vi "Lighting Test Software Lightshow.vi"() -> ()   [LabVIEW 2020]
panel:
  in  "Tab Control":enum32{"Map", "Settings", "LightShow"}(tab)=enum."LightShow"
  in  "Slide":dbl(slide)=0.7342857142857143 scale=0.0..1.0
  in  "Array 3":cluster{"Color Box":u32, "Slide":dbl}[][](array[cluster])=[[{"Color Box"=12303291, "Slide"=10.0}, {"Color Box"=12303291, "Slide"=10.0}, {"Color Box"=12303291, "Slide"=10.0}, {"Color Box"=12303291, "Slide"=10.0}, {"Color Box"=12303291, "Slide"=10.0}, {"Color Box"=12303291, "Slide"=10.0}], [{"Color Box"=12303291, "Slide"=10.0}, {"Color Box"=12303291, "Slide"=10.0}, {"Color Box"=12303291, "Slide"=10.0}, {"Color Box"=12303291, "Slide"=10.0}, {"Color Box"=12303291, "Slide"=10.0}, {"Color Box"=12303291, "Slide"=10.0}], [{"Color Box"=12303291, "Slide"=10.0}, {"Color Box"=12303291, "Slide"=10.0}, {"Color Box"=12303291, "Slide"=10.0}, {"Color Box"=12303291, "Slide"=10.0}, {"Color Box"=12303291, "Slide"=10.0}, {"Color Box"=12303291, "Slide"=10.0}], [{"Color Box"=12303291, "Slide"=10.0}, {"Color Box"=12303291, "Slide"=10.0}, {"Color Box"=12303291, "Slide"=10.0}, {"Color Box"=12303291, "Slide"=10.0}, {"Color Box"=0, "Slide"=0.0}, {"Color Box"=0, "Slide"=0.0}], [{"Color Box"=12303291, "Slide"=10.0}, {"Color Box"=12303291, "Slide"=10.0}, {"Color Box"=0, "Slide"=0.0}, {"Color Box"=12303291, "Slide"=10.0}, {"Color Box"=0, "Slide"=0.0}, {"Color Box"=0, "Slide"=0.0}], [{"Color Box"=0, "Slide"=0.0}, {"Color Box"=0, "Slide"=0.0}, {"Color Box"=12303291, "Slide"=10.0}, {"Color Box"=0, "Slide"=0.0}, {"Color Box"=0, "Slide"=0.0}, {"Color Box"=0, "Slide"=0.0}]] {"Slide" min=0.0 max=10.0 scale=-1.0..11.0 scale format="%_1g"}
  in  "Save Config":bool
  in  "Load Config":bool
  in  "Index":cluster{"Numeric":i32}[][](array[cluster])=[[{"Numeric"=3}, {"Numeric"=9}, {"Numeric"=2}, {"Numeric"=8}, {"Numeric"=19}, {"Numeric"=23}], [{"Numeric"=1}, {"Numeric"=11}, {"Numeric"=0}, {"Numeric"=10}, {"Numeric"=17}, {"Numeric"=21}], [{"Numeric"=5}, {"Numeric"=13}, {"Numeric"=4}, {"Numeric"=14}, {"Numeric"=27}, {"Numeric"=25}], [{"Numeric"=7}, {"Numeric"=15}, {"Numeric"=6}, {"Numeric"=12}, {"Numeric"=26}, {"Numeric"=24}], [{"Numeric"=29}, {"Numeric"=31}, {"Numeric"=-1}, {"Numeric"=18}, {"Numeric"=-1}, {"Numeric"=22}], [{"Numeric"=30}, {"Numeric"=-1}, {"Numeric"=16}, {"Numeric"=-1}, {"Numeric"=-1}, {"Numeric"=-1}]]
  in  "physical channels":refnum<k21>="Dev0/Ao0:15"
  in  "physical channels 2":refnum<k21>="Dev1/Ao0:15"
  out "error out":errorcluster
  out "specific error cleared?":bool
  in  "Choose Test":string(combo)="Test 1"
  out "Waveform Chart":dbl(graph)
  in  "LightShow":bool
  in  "OK":bool
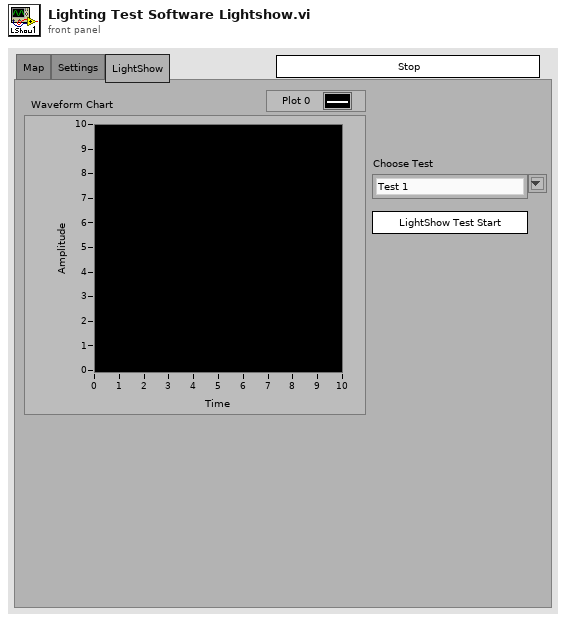
[diagram p1: front panel]
types:
  T1 = enum32{"invalid app kind", "Development System", "Run Time System", "Student Edition", "Embedded LabVIEW", "Evaluation", "Custom"}
  T2 = enum32{"Invalid", "Standard", "Closed", "Hidden", "Minimized", "Maximized"}
  T3 = cluster{"Slide Value Low":dbl, "Slide Value High":dbl}
  T4 = cluster{"Core":cluster{"Current VI Reference":refnum<vi>, "Close Panel on Exit?":bool}, "Your Boolean data":bool, "Slide Value":dbl, "Current Test":string, "Test Info":cluster{"Slide Value Low":dbl, "Slide Value High":dbl}}
  T5 = cluster{"Current VI Reference":refnum<vi>, "Close Panel on Exit?":bool}
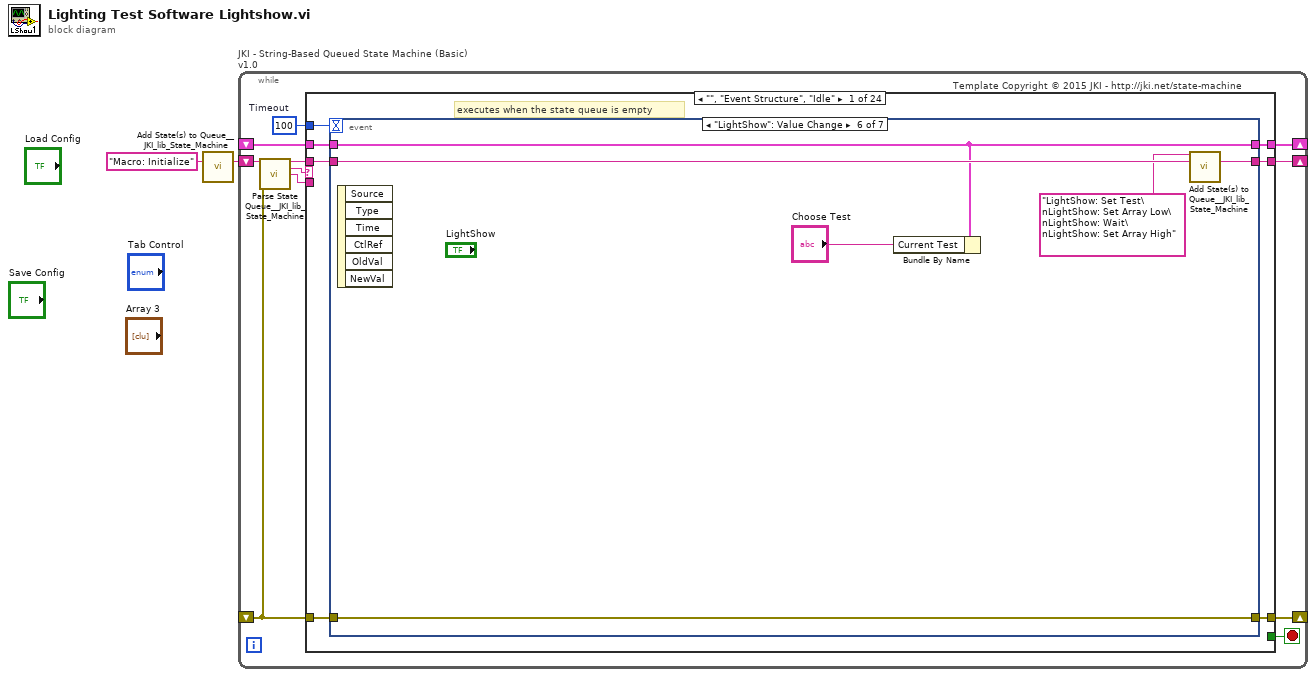
[diagram p0: block diagram]
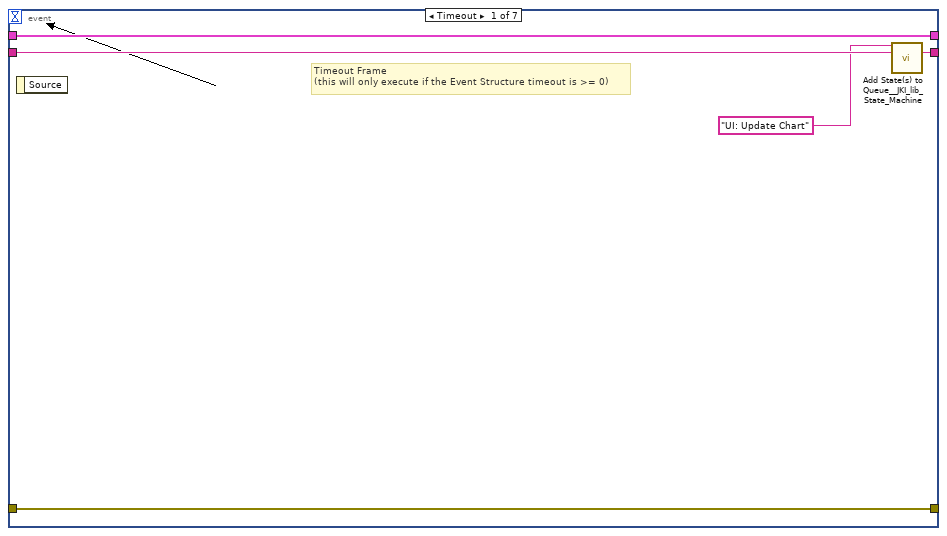
[diagram p2: hidden frame]
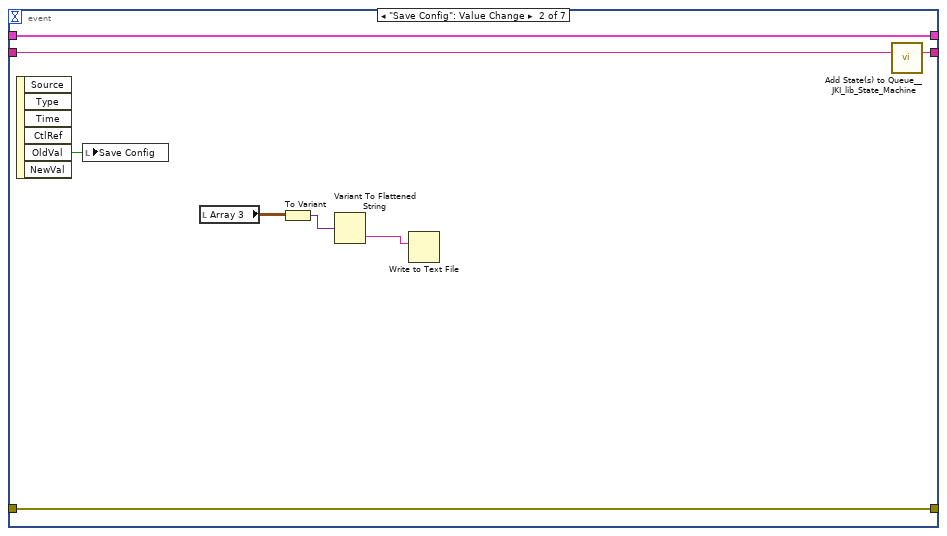
[diagram p3: hidden frame]
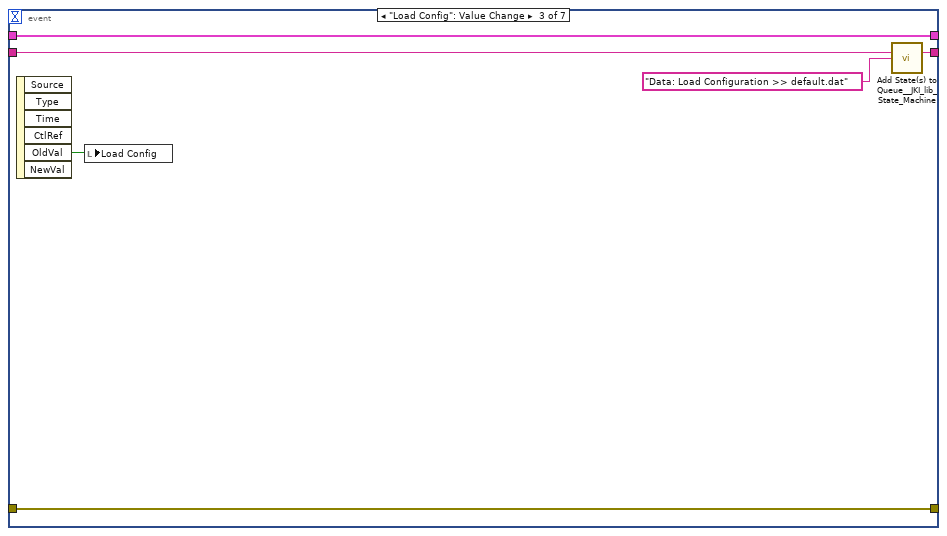
[diagram p4: hidden frame]
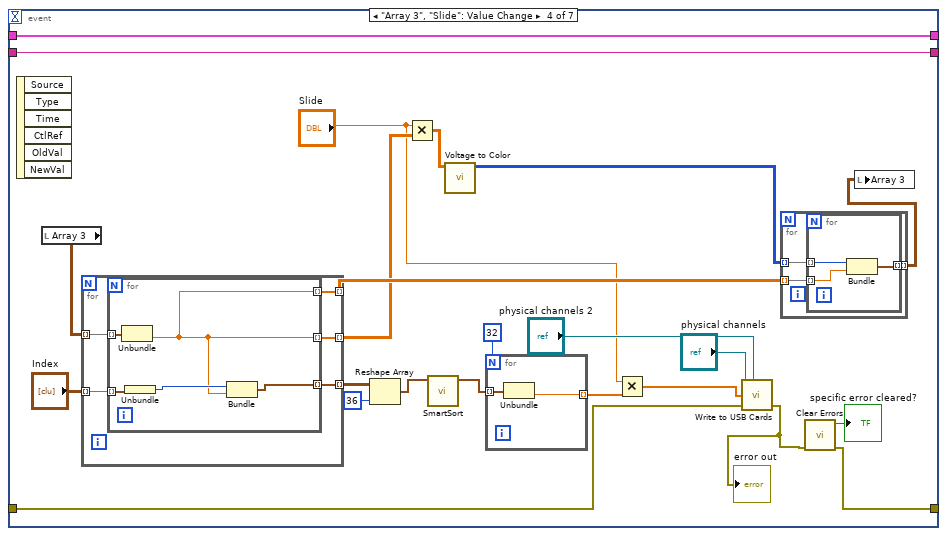
[diagram p5: hidden frame]
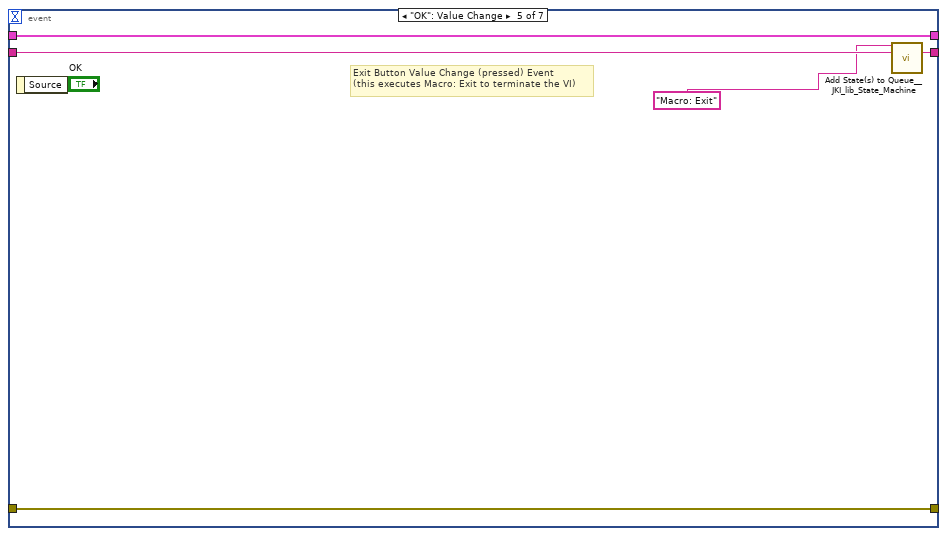
[diagram p6: hidden frame]
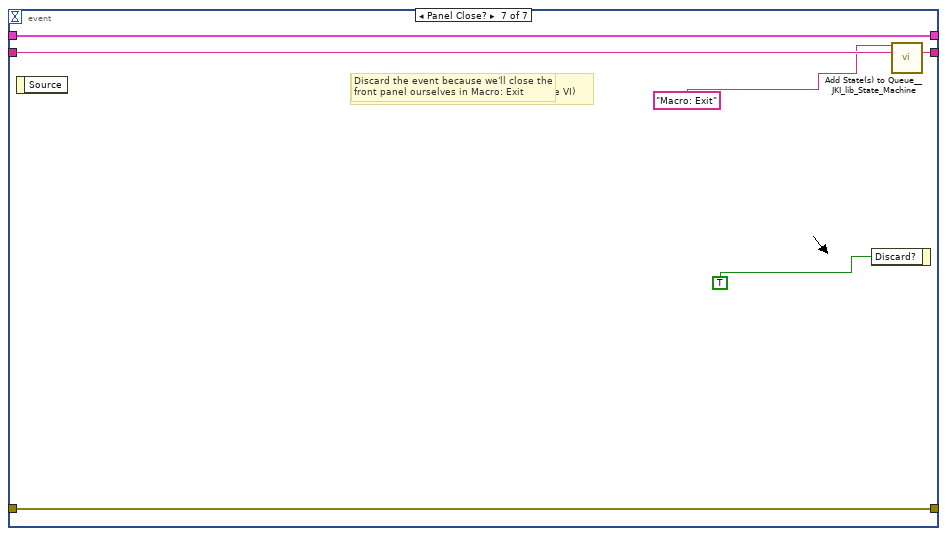
[diagram p7: hidden frame]
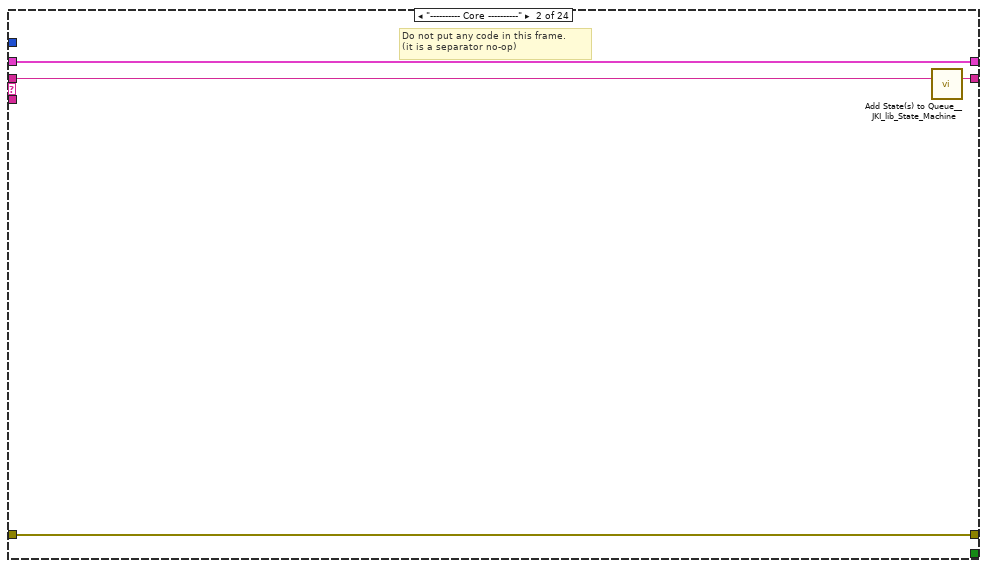
[diagram p8: hidden frame]
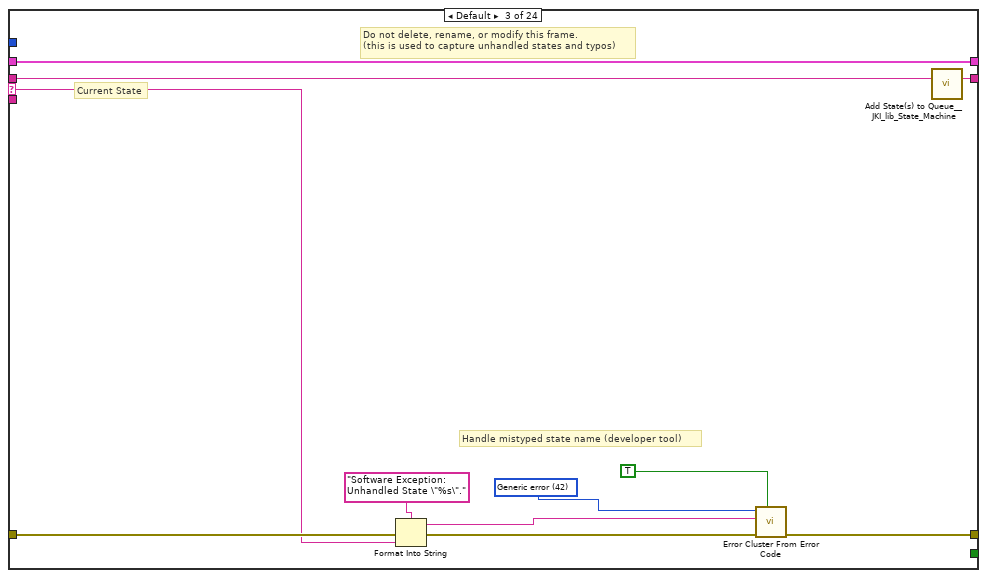
[diagram p9: hidden frame]
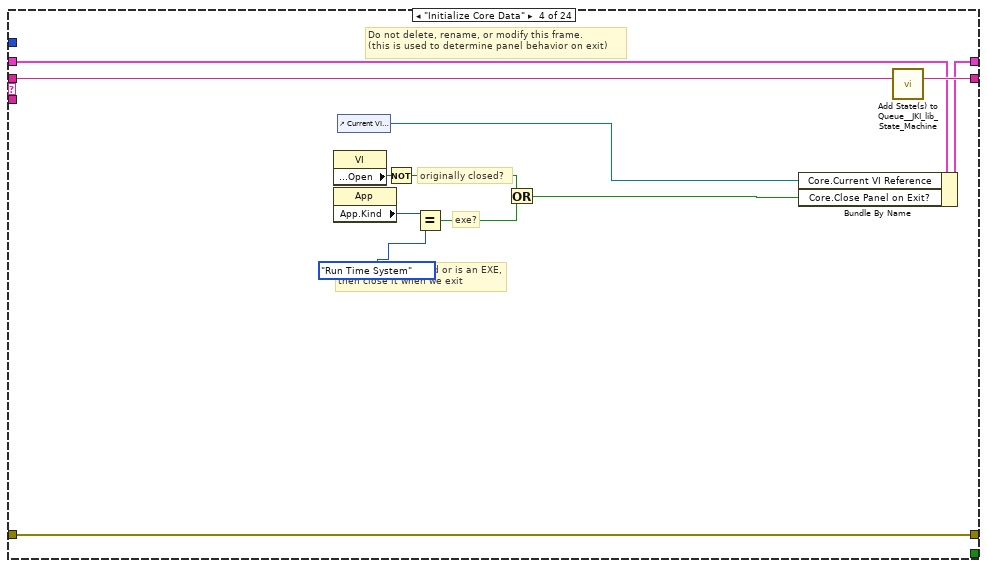
[diagram p10: hidden frame]
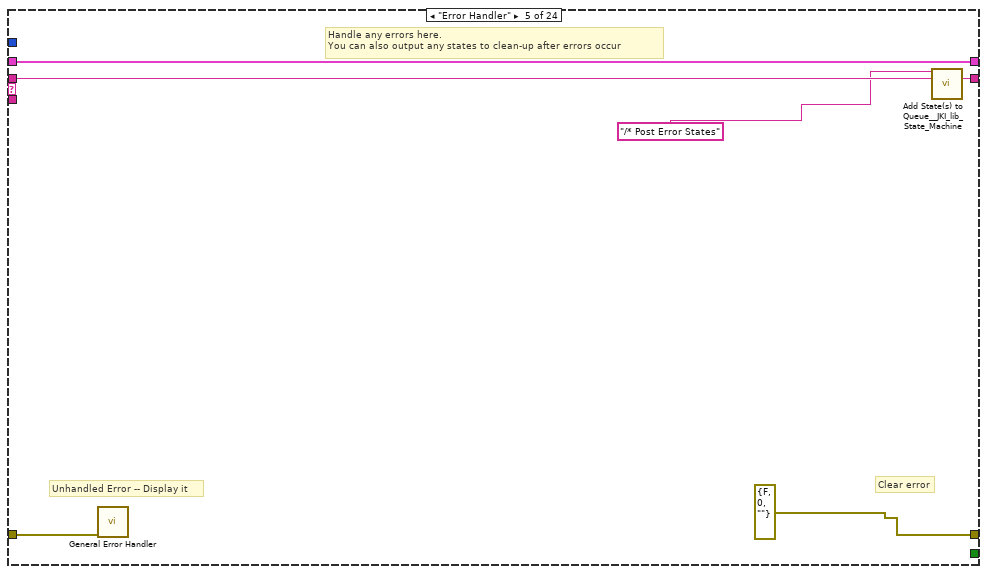
[diagram p11: hidden frame]
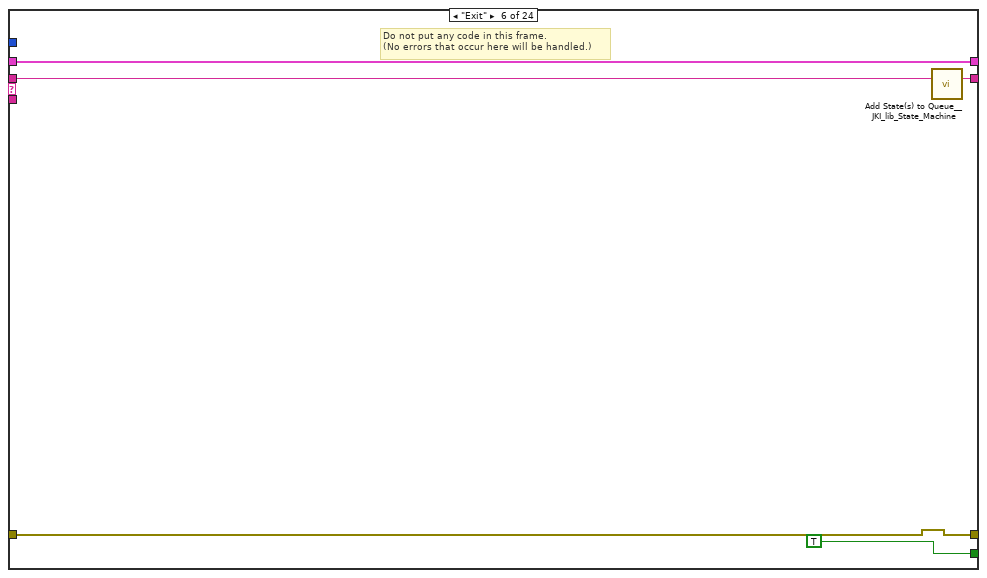
[diagram p12: hidden frame]
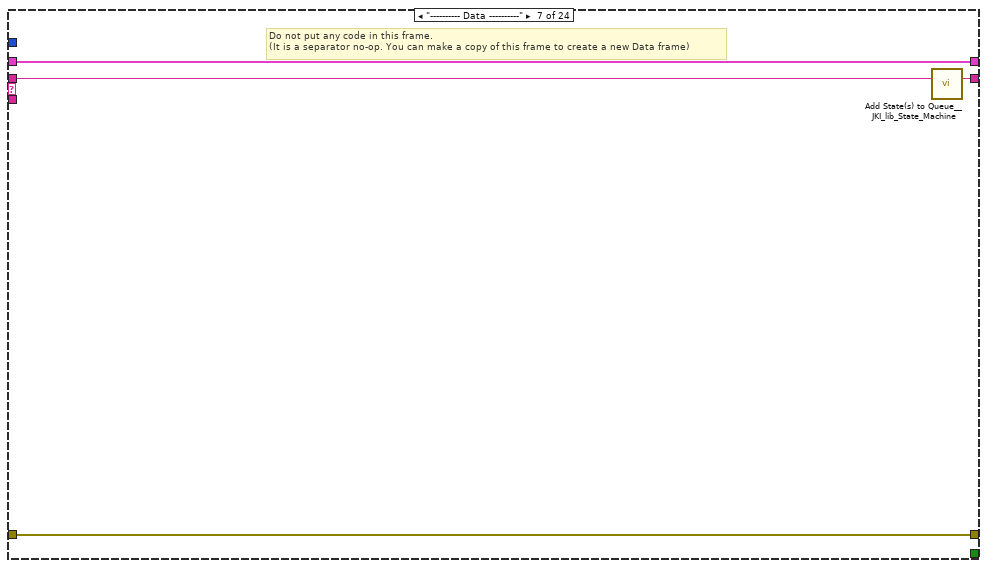
[diagram p13: hidden frame]
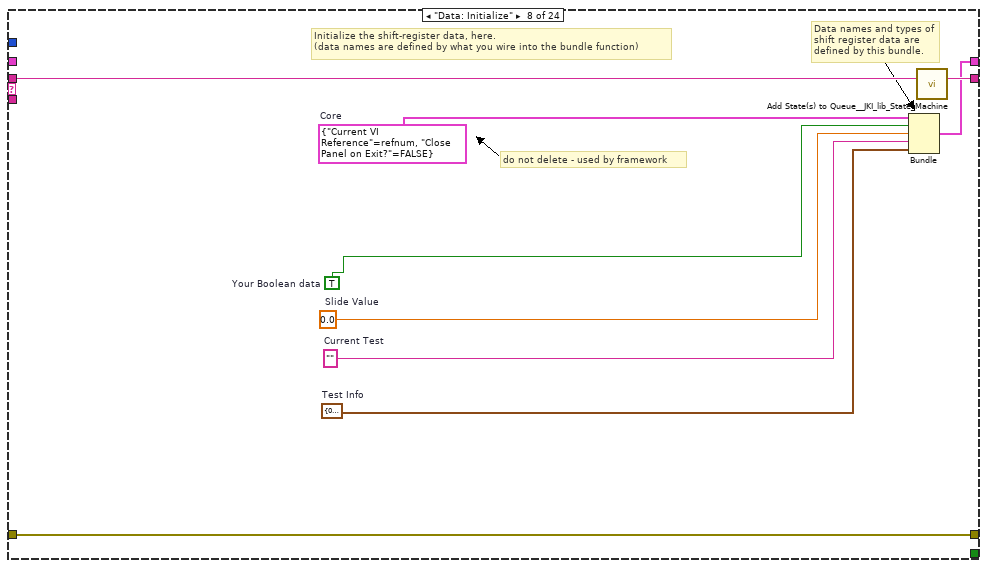
[diagram p14: hidden frame]
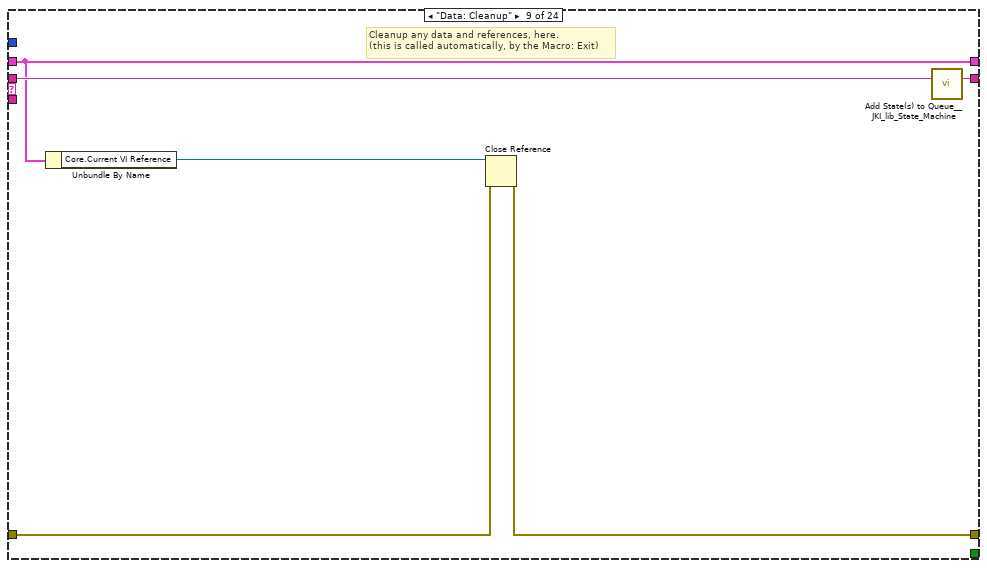
[diagram p15: hidden frame]
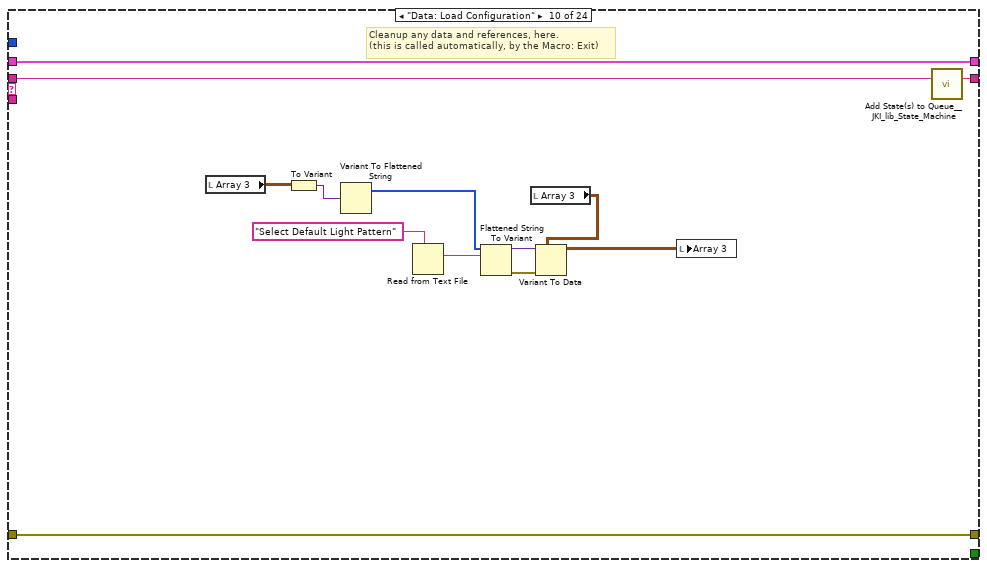
[diagram p16: hidden frame]
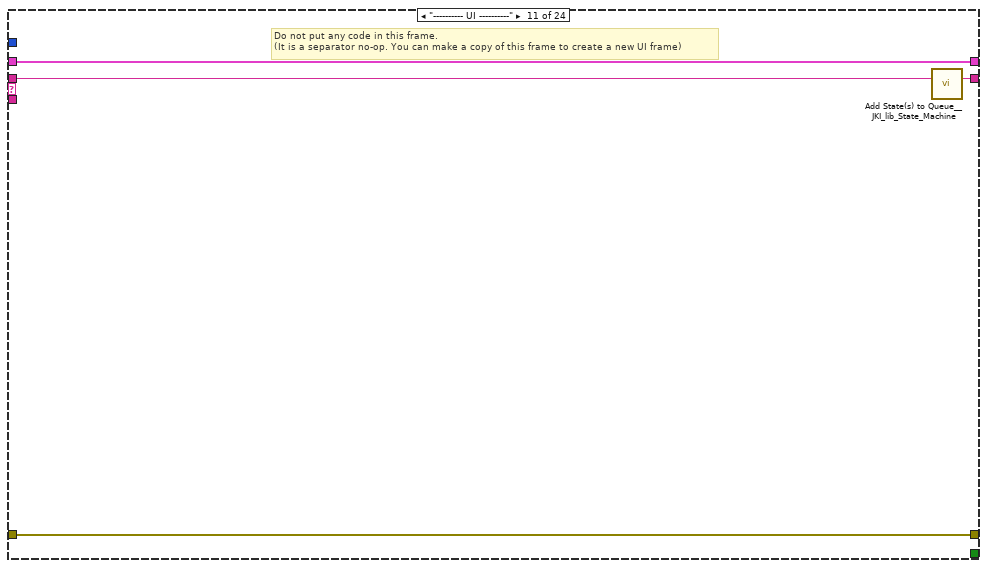
[diagram p17: hidden frame]
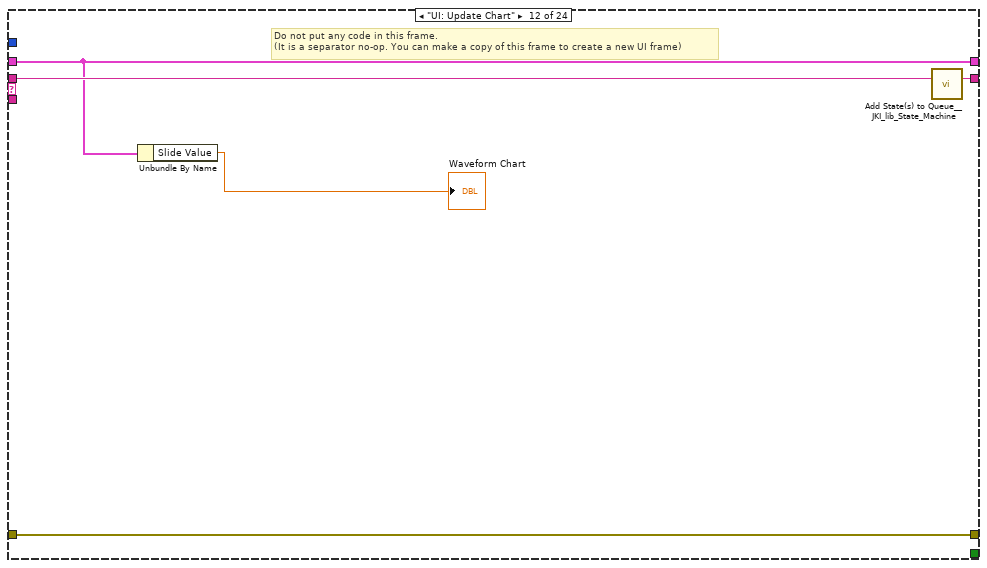
[diagram p18: hidden frame]
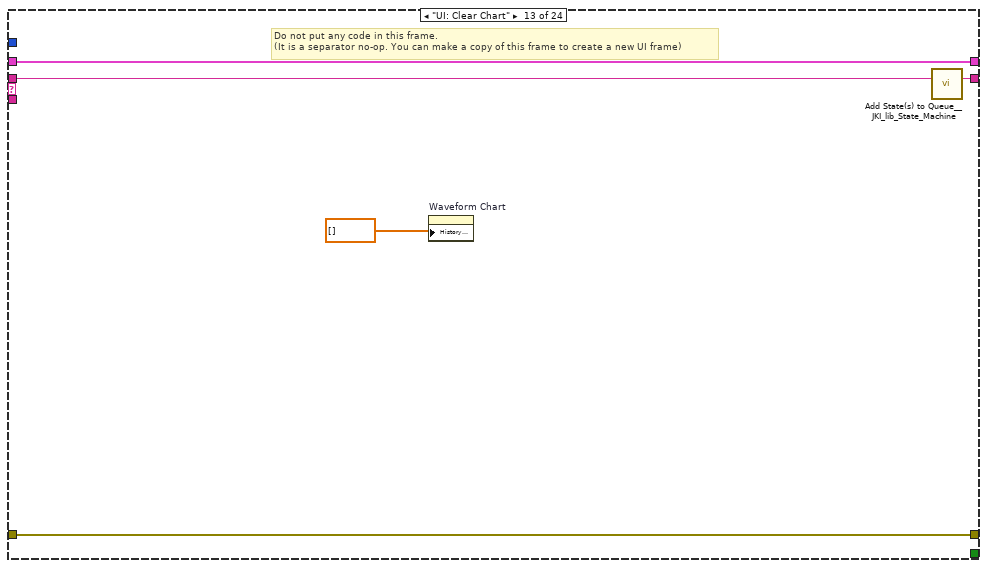
[diagram p19: hidden frame]
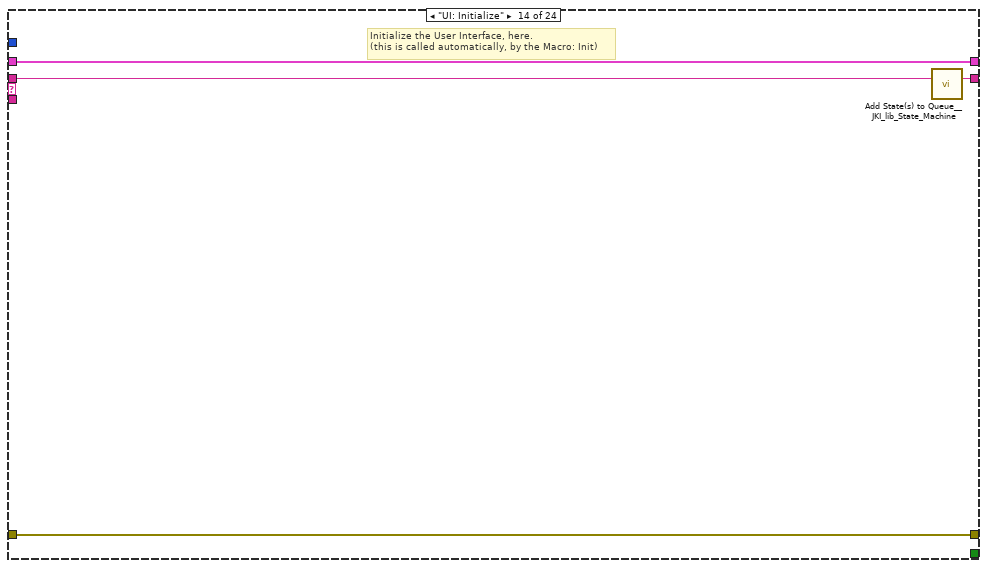
[diagram p20: hidden frame]
diagram:
  n1 = call <vilib>:"Add State(s) to Queue__JKI_lib_State_Machine.vi"("State(s) in (\"\")"="Macro: Initialize") -> ("States Out"=w2:string)  [unwired: 14 in]
  n2 = while "JKI - String-Based Queued State Machine (Basic) v1.0" {
    shift-right: [w6] -> _
    shift-left: _ -> [w5]
    shift-right: [w9] -> _
    shift-left: _ -> [w3]
    shift-right: [w8] -> _
    shift-left: w2 -> [w10]
    stop <- w7 stop-if-true
    w4 = 100  # Timeout
    # "Template Copyright © 2015 JKI - http://jki.net/state-machine"
    n3 = call <vilib>:"Parse State Queue__JKI_lib_State_Machine.vi"("State Queue"=w10, "Error In (no error)"=w3) -> ("Remaining States"=w12:string, "Current State"=w13:string, "Arguments"=w11:string)  [unwired: 11 in]
    n4 = case shown="\"\", \"Event Structure\", \"Idle\"" w13 {
      selector: w13 -> [_ _ w102 _ _ _ _ _ _ _ _ _ _ _ _ _ _ _ _ _ _ _ _ _]
      tunnel: w12 -> [w20 w101 w106 w124 w130 w135 w139 w148 w154 w167 w171 w176 w181 w185 w191 w202 w228 w233 w243 w247 w255 w262 w290 w333]
      tunnel: w11 -> [_ _ _ _ _ _ _ _ _ _ _ _ _ _ w186 w196 _ _ _ _ _ _ _ _]
      tunnel: w5 -> [w18 w98 w104 w115 w127 w132 w136 _ w149 w165 w168 w173 w178 w183 w189 w198 w225 w230 w240 w244 w253 w257 w268 w311]
      tunnel: [w17 w99 w108 w121 errorcluster {"status"=FALSE, "code"=0, "source"=""} ("error out") w131 w137 w143 w150 w164 w169 w174 w179 w182 w187 w199 w226 w231 w241 w245 w251 w260 w269 w312] -> w9
      tunnel: w3 -> [w16 w99 w107 w121 w126 w131 w137 w143 w151 w164 w169 w174 w179 w182 w188 w200 w226 w231 w241 w245 w252 w260 w270 w313]
      tunnel: [w19 w100 w105 w123 w129 w134 w138 w147 w153 w166 w170 w175 w180 w184 w190 w201 w227 w232 w242 w246 w254 w261 w289 w332] -> w8
      tunnel: [_ _ _ _ _ TRUE _ _ _ _ _ _ _ _ _ _ _ _ _ _ _ _ _ _] -> w7
      tunnel: [w15 w98 w104 w122 w127 w132 w136 w146 w149 w165 w168 w173 w178 w183 w189 w198 w225 w230 w240 w244 w253 w257 w267 w310] -> w6
      tunnel: w4 -> [w14 _ _ _ _ _ _ _ _ _ _ _ _ _ _ _ _ _ _ _ _ _ _ _]
      frame "", "Event Structure", "Idle" {
        # "executes when the state queue is empty"
        n5 = event shown="[5] \"LightShow\": Value Change" {
          selector: _ -> [_ _ _ _ _ _ _]
          dyn-events: _ -> [_ _ _ _ _ _ _]
          timeout: w14 -> [_ _ _ _ _ _ _]
          tunnel: w20 -> [w25 w33 w39 w61 w85 w90 w97]
          tunnel: [w24 w32 w38 w61 w84 w91 w96] -> w19
          tunnel: w18 -> [w22 w30 w36 w62 w82 w88 w94]
          tunnel: [w23 w31 w37 w47 w83 w86 w95] -> w17
          tunnel: w16 -> [w23 w31 w37 w48 w83 w86 w95]
          tunnel: [w22 w30 w36 w62 w82 w88 w94] -> w15
          event Timeout {
            # "Timeout Frame\n(this will only execute if the Event Structure timeout is >= 0)"
            n6 = event-data() -> ()  [unwired: 1 in, 1 out]
            n7 = call <vilib>:"Add State(s) to Queue__JKI_lib_State_Machine.vi"("State(s) in Front (\"\")"="UI: Update Chart" ("State(s) in Front (\"\")"), "State(s) in (\"\")"=w25) -> ("States Out"=w24:string)  [unwired: 13 in]
          }
          event "Save Config": Value Change {
            n8 = event-data() -> ("OldVal"=w26:bool)  [unwired: 1 in, 5 out]
            n9 = local write "Save Config"(w26) -> ()
            n10 = local read "Array 3"() -> (w29:cluster{"Color Box":u32, "Slide":dbl}[][])
            n11 = To Variant(anything=w29) -> (Variant=w28:variant)
            n12 = Variant To Flattened String(Variant=w28) -> (data string=w27:string)  [unwired: 1 out]
            n13 = Write to Text File(text=w27) -> ()  [unwired: 3 in, 3 out]
            n14 = call <vilib>:"Add State(s) to Queue__JKI_lib_State_Machine.vi"("State(s) in (\"\")"=w33) -> ("States Out"=w32:string)  [unwired: 14 in]
          }
          event "Load Config": Value Change {
            n15 = event-data() -> ("OldVal"=w35:bool)  [unwired: 1 in, 5 out]
            n16 = local write "Load Config"(w35) -> ()
            n17 = call <vilib>:"Add State(s) to Queue__JKI_lib_State_Machine.vi"("State(s) in (\"\")"=w39, "State(s) at Back (\"\")"="Data: Load Configuration >> default.dat") -> ("States Out"=w38:string)  [unwired: 13 in]
          }
          event "Array 3", "Slide": Value Change {
            n18 = event-data() -> ()  [unwired: 1 in, 6 out]
            n19 = local read "Array 3"() -> (w60:cluster{"Color Box":u32, "Slide":dbl}[][])
            n20 = for {
              tunnel: w60 -> [w75] mode=indexing
              tunnel: [w74] -> w44 mode=indexing
              tunnel: [w73] -> w57 mode=indexing
              tunnel: "Index" -> [w72] mode=indexing
              tunnel: [w71] -> w55 mode=indexing
              n21 = for {
                tunnel: w75 -> [w80] mode=indexing
                tunnel: [w77] -> w74 mode=indexing
                tunnel: [w77] -> w73 mode=indexing
                tunnel: w72 -> [w79] mode=indexing
                tunnel: [w76] -> w71 mode=indexing
                n22 = Unbundle(w80) -> ("Slide"=w77:dbl)  [unwired: 1 out]
                n23 = Unbundle(w79) -> ("Numeric"=w78:i32)
                n24 = Bundle("Numeric"=w78, "Slide"=w77) -> (w76:cluster{"Numeric":i32, "Slide":dbl})  [unwired: 1 in]
              }
            }
            n25 = Reshape Array(w55, 36 ("dimension size")) -> (w53:cluster{"Numeric":i32, "Slide":dbl}[])
            n26 = Multiply(x="Slide", y=w44) -> (x*y=w43:dbl[][])
            n27 = call "SmartSort.vi"("Array in"=w53) -> ("Array out"=w52:cluster{"Numeric":i32, "Slide":dbl}[])  [unwired: 10 in]
            n28 = call "Voltage to Color.vi"("Array in"=w43) -> ("Array out"=w58:u32[][])  [unwired: 10 in]
            n29 = for {
              N: 32 -> [_]
              tunnel: w52 -> [w64] mode=indexing
              tunnel: [w63] -> w42 mode=indexing
              n30 = Unbundle(w64) -> ("Slide"=w63:dbl)  [unwired: 1 out]
            }
            n31 = Multiply(x="Slide", y=w42) -> (x*y=w40:dbl[])
            n32 = call "Write to USB Cards.vi"("physical channels"="physical channels", "physical channels 2"="physical channels 2", "Array"=w40, "error in"=w48) -> ("error out"=w45:errorcluster)  [unwired: 5 in]
            "error out" <- w45
            n33 = for {
              tunnel: [w67] -> w59 mode=indexing
              tunnel: w58 -> [w66] mode=indexing
              tunnel: w57 -> [w65] mode=indexing
              n34 = for {
                tunnel: [w70] -> w67 mode=indexing
                tunnel: w66 -> [w69] mode=indexing
                tunnel: w65 -> [w68] mode=indexing
                n35 = Bundle(w69, "Slide"=w68) -> (w70:cluster{u32, "Slide":dbl})  [unwired: 1 in]
              }
            }
            n36 = call <vilib>:"Clear Errors.vi"("error in (no error)"=w45) -> ("error out"=w47:errorcluster, "specific error cleared?"=→"specific error cleared?":bool)  [unwired: 5 in]
            n37 = local write "Array 3"(w59) -> ()
          }
          event "OK": Value Change {
            # "Exit Button Value Change (pressed) Event\n(this executes Macro: Exit to terminate the VI)"
            n38 = event-data() -> ()  [unwired: 1 in, 1 out]
            n39 = call <vilib>:"Add State(s) to Queue__JKI_lib_State_Machine.vi"("State(s) in Front (\"\")"="Macro: Exit", "State(s) in (\"\")"=w85) -> ("States Out"=w84:string)  [unwired: 13 in]
          }
          event "LightShow": Value Change {
            n40 = event-data() -> ()  [unwired: 1 in, 6 out]
            n41 = Bundle By Name(cluster=w88, "Current Test"="Choose Test") -> ()  [unwired: 1 out]
            n42 = call <vilib>:"Add State(s) to Queue__JKI_lib_State_Machine.vi"("State(s) in Front (\"\")"="LightShow: Set Test\nLightShow: Set Array Low\nLightShow: Wait\nLightShow: Set Array High" ("State(s) in Front (\"\")"), "State(s) in (\"\")"=w90) -> ("States Out"=w91:string)  [unwired: 13 in]
          }
          event Panel Close? {
            # "Discard the event because we'll close the front panel ourselves in Macro: Exit"
            # "Close Panel button (pressed) Event\n(this executes Macro: Exit to terminate the VI)"
            n43 = event-data() -> ()  [unwired: 1 in, 1 out]
            n44 = event-data("Discard?"=TRUE) -> ()  [unwired: 1 in, 1 out]
            n45 = call <vilib>:"Add State(s) to Queue__JKI_lib_State_Machine.vi"("State(s) in Front (\"\")"="Macro: Exit", "State(s) in (\"\")"=w97) -> ("States Out"=w96:string)  [unwired: 13 in]
          }
        }
      }
      frame "---------- Core ----------" {
        # "Do not put any code in this frame.\n(it is a separator no-op)"
        n46 = call <vilib>:"Add State(s) to Queue__JKI_lib_State_Machine.vi"("State(s) in (\"\")"=w101) -> ("States Out"=w100:string)  [unwired: 14 in]
      }
      frame Default {
        w111 = 42 items=["No error", "Argument error", "Memory is full", "Out of zone", "End of file", "File already open", "Generic file I/O error", "File not found", "File permission error", "Disk is full", "Duplicate path", "Too many files open", "System feature not enabled", "Resource file not found", "Cannot add resource", "Resource not found", "Image not found", "Image memory error", "Pen does not exist", "Config type invalid", "Config token not found", "Config parse error", "Config memory error", "Bad external code format", "Bad external code offset", "External code not present", "Null window", "Destroy window error", "Null menu", "Print aborted", "Bad print record", "Print driver error", "Windows error during printing", "Memory error during printing", "Print dialog error", "Generic print error", "Invalid device refnum", "Device not found", "Device parameter error", "Device unit error", "Cannot open device", "Device call aborted", "Generic error", "Cancelled by user", "Object ID too low", "Object ID too high", "Object not in heap", "Unknown heap", "Unknown object (invalid DefProc)", "Unknown object (DefProc not in table)", "Message out of range", "Invalid (null) method", "Unknown message", "Manager call not supported", "Bad address", "Network operation in progress", "Network operation timed out", "Connection is busy", "Network attribute not supported", "Network error", "Address in use", "System out of memory", "Connection aborted", "Connection refused", "Not connected", "Already connected", "Connection closed", "Initialization error (interapplication manager)", "Bad occurrence", "Wait on unbound occurrence handler", "Occurrence queue overflow", "Datalog type conflict", "Unused", "Unrecognized type (interapplication manager)", "Memory corrupt", "Failed to make temporary DLL", "Old CIN version", "Drag socket not found", "Failed to load drop-object", "Failed to register OLE object", "Failed to release OLE object", "Format specifier type mismatch", "Unknown format specifier", "Too few format specifiers", "Too many format specifiers", "Scan failed", "Newer CIN version", "Error converting to variant", "Runtime menu error", "Password tampered", "Variant attribute not found", "Incompatible variant data type", "Event data is not available", "Event Store is not present", "Occurrence is not found", "Event Queue is not created", "Event info is not available", "Refnum passed is NULL", "Error retrieving Class GUID", "Error retrieving CoClass GUID", "Error retrieving TypeLib GUID.", "Bad built application magic bytes.", "Specific driver is different from the specific driver associated with the Logical Name.", "There is no session opened to the class driver.", "Max Error", "MAX - Error with config objects", "MAX - Error loading configuration", "MAX - Group not supported"]
        # "Current State"
        # "Do not delete, rename, or modify this frame.\n(this is used to capture unhandled states and typos)"
        # "Handle mistyped state name (developer tool)"
        n47 = Format Into String(format string="Software Exception: Unhandled State \"%s\"." ("message"), error in=w107, w102) -> (resulting string=w110:string, error out=w109:errorcluster)  [unwired: 1 in]
        n48 = call <vilib>:"Error Cluster From Error Code.vi"("show call chain? (False)"=TRUE, "error in (no error)"=w109, "error message (\"\")"=w110, "error code (0)"=w111) -> ("error out"=w108:errorcluster)  [unwired: 5 in]
        n49 = call <vilib>:"Add State(s) to Queue__JKI_lib_State_Machine.vi"("State(s) in (\"\")"=w106) -> ("States Out"=w105:string)  [unwired: 14 in]
      }
      frame "Initialize Core Data" {
        # "Do not delete, rename, or modify this frame.\n(this is used to determine panel behavior on exit)"
        # "originally closed?"
        # "exe?"
        # "If panel starts closed or is an EXE, then close it when we exit"
        n50 = property class="VI"() -> ("Front Panel.Open"=w120:bool)  [unwired: 2 in, 2 out]
        n51 = property class="App"() -> ("App.Kind"=w119:T1)  [unwired: 2 in, 2 out]
        n52 = control-ref of="Current VI Reference"() -> (w113:refnum<vi>)
        n53 = Not(x=w120) -> (.not. x?=w117:bool)
        n54 = Equal?(x=w119, y=T1."Run Time System" ("Application:Kind")) -> (x = y?=w116:bool)
        n55 = Or(x=w117, y=w116) -> (x .or. y?=w114:bool)
        n56 = Bundle By Name(cluster=w115, "Core.Current VI Reference"=w113, "Core.Close Panel on Exit?"=w114) -> (w122:T4)
        n57 = call <vilib>:"Add State(s) to Queue__JKI_lib_State_Machine.vi"("State(s) in (\"\")"=w124) -> ("States Out"=w123:string)  [unwired: 14 in]
      }
      frame "Error Handler" {
        # "Unhandled Error -- Display it"
        # "Handle any errors here.\nYou can also output any states to clean-up after errors occur"
        # "Clear error"
        n58 = call <vilib>:"General Error Handler.vi"("error in (no error)"=w126) -> ()  [unwired: 10 in, 5 out]
        n59 = call <vilib>:"Add State(s) to Queue__JKI_lib_State_Machine.vi"("State(s) in Front (\"\")"="/* Post Error States", "State(s) in (\"\")"=w130) -> ("States Out"=w129:string)  [unwired: 13 in]
      }
      frame "Exit" {
        # "Do not put any code in this frame.\n(No errors that occur here will be handled.)"
        n60 = call <vilib>:"Add State(s) to Queue__JKI_lib_State_Machine.vi"("State(s) in (\"\")"=w135) -> ("States Out"=w134:string)  [unwired: 14 in]
      }
      frame "---------- Data ----------" {
        # "Do not put any code in this frame.\n(It is a separator no-op. You can make a copy of this frame to create a new Data frame)"
        n61 = call <vilib>:"Add State(s) to Queue__JKI_lib_State_Machine.vi"("State(s) in (\"\")"=w139) -> ("States Out"=w138:string)  [unwired: 14 in]
      }
      frame "Data: Initialize" {
        w140 = T3 {"Slide Value Low"=0.0, "Slide Value High"=0.0}  # Test Info
        w141 = ""  # Current Test
        w142 = 0.0  # Slide Value
        w144 = T5 {"Current VI Reference"=refnum, "Close Panel on Exit?"=FALSE}  # Core
        w145 = TRUE  # Your Boolean data
        # "do not delete - used by framework"
        # "Data names and types of shift register data are defined by this bundle."
        # "Initialize the shift-register data, here.\n(data names are defined by what you wire into the bundle function)"
        n62 = Bundle("Core"=w144, "Your Boolean data"=w145, "Slide Value"=w142, "Current Test"=w141, "Test Info"=w140) -> (w146:T4)  [unwired: 1 in]
        n63 = call <vilib>:"Add State(s) to Queue__JKI_lib_State_Machine.vi"("State(s) in (\"\")"=w148) -> ("States Out"=w147:string)  [unwired: 14 in]
      }
      frame "Data: Cleanup" {
        # "Cleanup any data and references, here.\n(this is called automatically, by the Macro: Exit)"
        n64 = Unbundle By Name(w149) -> ("Core.Current VI Reference"=w152:refnum<vi>)
        n65 = Close Reference(reference=w152, error in (no error)=w151) -> (error out=w150:errorcluster)
        n66 = call <vilib>:"Add State(s) to Queue__JKI_lib_State_Machine.vi"("State(s) in (\"\")"=w154) -> ("States Out"=w153:string)  [unwired: 14 in]
      }
      frame "Data: Load Configuration" {
        # "Cleanup any data and references, here.\n(this is called automatically, by the Macro: Exit)"
        n67 = local read "Array 3"() -> (w163:cluster{"Color Box":u32, "Slide":dbl}[][])
        n68 = To Variant(anything=w163) -> (Variant=w158:variant)
        n69 = Variant To Flattened String(Variant=w158) -> (1:w161:i16[])  [unwired: 1 out]
        n70 = Read from Text File(prompt (Open existing file)="Select Default Light Pattern") -> (text=w162:string)  [unwired: 3 in, 3 out]
        n71 = Flattened String To Variant(6:w162, 7:w161) -> (0:w160:errorcluster, 3:w159:variant)  [unwired: 1 in]
        n72 = local read "Array 3"() -> (w156:cluster{"Color Box":u32, "Slide":dbl}[][])
        n73 = Variant To Data(error in=w160, type=w156, Variant=w159) -> (data=w157:cluster{"Color Box":u32, "Slide":dbl}[][])  [unwired: 1 out]
        n74 = local write "Array 3"(w157) -> ()
        n75 = call <vilib>:"Add State(s) to Queue__JKI_lib_State_Machine.vi"("State(s) in (\"\")"=w167) -> ("States Out"=w166:string)  [unwired: 14 in]
      }
      frame "---------- UI ----------" {
        # "Do not put any code in this frame.\n(It is a separator no-op. You can make a copy of this frame to create a new UI frame)"
        n76 = call <vilib>:"Add State(s) to Queue__JKI_lib_State_Machine.vi"("State(s) in (\"\")"=w171) -> ("States Out"=w170:string)  [unwired: 14 in]
      }
      frame "UI: Update Chart" {
        # "Do not put any code in this frame.\n(It is a separator no-op. You can make a copy of this frame to create a new UI frame)"
        n77 = Unbundle By Name(w173) -> ("Slide Value"=→"Waveform Chart":dbl)
        n78 = call <vilib>:"Add State(s) to Queue__JKI_lib_State_Machine.vi"("State(s) in (\"\")"=w176) -> ("States Out"=w175:string)  [unwired: 14 in]
      }
      frame "UI: Clear Chart" {
        # "Do not put any code in this frame.\n(It is a separator no-op. You can make a copy of this frame to create a new UI frame)"
        n79 = property on="Waveform Chart" class="WFChart (strict)"("History Data"=dbl[] []) -> ()  [unwired: 2 in, 2 out]
        n80 = call <vilib>:"Add State(s) to Queue__JKI_lib_State_Machine.vi"("State(s) in (\"\")"=w181) -> ("States Out"=w180:string)  [unwired: 14 in]
      }
      frame "UI: Initialize" {
        # "Initialize the User Interface, here.\n(this is called automatically, by the Macro: Init)"
        n81 = call <vilib>:"Add State(s) to Queue__JKI_lib_State_Machine.vi"("State(s) in (\"\")"=w185) -> ("States Out"=w184:string)  [unwired: 14 in]
      }
      frame "UI: Cursor Set" {
        # "Argument"
        # "Set and Unset Cursor Busy.\n(Usage: \"UI: Cursor Set >> Busy|Idle\")"
        n82 = case shown="\"Idle\", Default" w186 {
          tunnel: w188 -> [w193 w195]
          tunnel: [w192 w194] -> w187
          frame "Idle", Default {
            n83 = call <vilib>:"Unset Busy.vi"("error in (no error)"=w193) -> ("error out"=w192:errorcluster)  [unwired: 10 in]
          }
          frame "Busy" {
            n84 = call <vilib>:"Set Busy.vi"("error in (no error)"=w195) -> ("error out"=w194:errorcluster)  [unwired: 9 in, 1 out]
          }
        }
        n85 = call <vilib>:"Add State(s) to Queue__JKI_lib_State_Machine.vi"("State(s) in (\"\")"=w191) -> ("States Out"=w190:string)  [unwired: 14 in]
      }
      frame "UI: Front Panel State" {
        # "Argument"
        # "Set Front Panel Open or Closed\n(Usage: \"UI: Front Panel State >> Open|Close\")"
        n86 = Unbundle By Name(w198) -> ("Core.Current VI Reference"=w197:refnum<vi>)
        n87 = case shown="\"Open\", Default" w196 {
          tunnel: w200 -> [w206 w219]
          tunnel: [w208 w220] -> w199
          tunnel: w197 -> [w207 w217]
          frame "Open", Default {
            n88 = property class="VI"(reference=w207, error in=w206) -> (reference out=w204:refnum<vi>, error out=w205:errorcluster, "Front Panel.Open"=w203:bool)
            n89 = case shown="False" w203 {
              tunnel: [w211 w214] -> w208
              tunnel: w205 -> [w210 w214]
              tunnel: w204 -> [w209 _]
              frame False {
                n90 = invoke class="VI" method="FP.Open"(reference=w209, error in=w210, "Activate"=TRUE, "State"=T2."Standard") -> (error out=w211:errorcluster)  [unwired: 1 in, 4 out]
              }
              frame True {
              }
            }
          }
          frame "Close" {
            n91 = property class="VI"(reference=w217, error in=w219) -> (reference out=w216:refnum<vi>, error out=w218:errorcluster, "Front Panel.Open"=w215:bool)
            n92 = case shown="True" w215 {
              tunnel: [w221 w224] -> w220
              tunnel: w218 -> [w221 w223]
              tunnel: w216 -> [_ w222]
              frame False {
              }
              frame True {
                n93 = invoke class="VI" method="FP.Close"(reference=w222, error in=w223) -> (error out=w224:errorcluster)  [unwired: 1 in, 2 out]
              }
            }
          }
        }
        n94 = call <vilib>:"Add State(s) to Queue__JKI_lib_State_Machine.vi"("State(s) in (\"\")"=w202) -> ("States Out"=w201:string)  [unwired: 14 in]
      }
      frame "---------- Macro ----------" {
        # "Do not put any code in this frame.\n(It is a separator no-op. You can make a copy of this frame to create a new Macro frame)"
        n95 = call <vilib>:"Add State(s) to Queue__JKI_lib_State_Machine.vi"("State(s) in (\"\")"=w228) -> ("States Out"=w227:string)  [unwired: 14 in]
      }
      frame "Macro: Initialize" {
        w229 = "Data: Initialize\nInitialize Core Data\nUI: Initialize\nUI: Clear Chart\nUI: Front Panel State >> Open"  # Data: Initialize Initialize Core Data UI: Initialize UI: Clear Chart UI: Front Panel State >> Open
        # "Initialization Macro\n(This is called once, when the VI starts)"
        n96 = call <vilib>:"Add State(s) to Queue__JKI_lib_State_Machine.vi"("State(s) in Front (\"\")"=w229, "State(s) in (\"\")"=w233) -> ("States Out"=w232:string)  [unwired: 13 in]
      }
      frame "Macro: Exit" {
        # "Exit Macro\n(This is called once, when the VI exits)"
        n97 = Unbundle By Name(w240) -> ("Core.Close Panel on Exit?"=w239:bool)
        n98 = Select(t="UI: Front Panel State >> Close", s=w239, f="") -> (s? t:f=w236:string)
        n99 = call <vilib>:"Add State(s) to Queue__JKI_lib_State_Machine.vi"("State(s) in (\"\")"=w236, "State(s) at Back (\"\")"="Data: Cleanup\nExit") -> ("States Out"=w234:string)  [unwired: 13 in]
        n100 = call <vilib>:"Add State(s) to Queue__JKI_lib_State_Machine.vi"("State(s) in Front (\"\")"=w234, "State(s) in (\"\")"=w243) -> ("States Out"=w242:string)  [unwired: 13 in]
      }
      frame "---------- LightShow ----------" {
        # "Template Separator\n(You can make a copy of, or modify, this frame)"
        n101 = call <vilib>:"Add State(s) to Queue__JKI_lib_State_Machine.vi"("State(s) in (\"\")"=w247) -> ("States Out"=w246:string)  [unwired: 14 in]
      }
      frame "LightShow: Wait" {
        # "Template Separator\n(You can make a copy of, or modify, this frame)"
        n102 = Multiply(x=5.0, y=1000.0) -> (x*y=w248:dbl)
        n103 = call <userlib>:"Wait (ms)__ogtk.vi"("error in (no error)"=w252, "milliseconds to wait"=w248) -> ("error out"=w251:errorcluster)  [unwired: 8 in, 1 out]
        n104 = call <vilib>:"Add State(s) to Queue__JKI_lib_State_Machine.vi"("State(s) in (\"\")"=w255) -> ("States Out"=w254:string)  [unwired: 14 in]
      }
      frame "LightShow: Set Test" {
        # "Template Separator\n(You can make a copy of, or modify, this frame)"
        n105 = Unbundle By Name(w257) -> ("Current Test"=w259:string)
        n106 = Decimal String To Number(string=w259) -> (number=w258:i32)  [unwired: 2 in, 1 out]
        n107 = case shown="3" w258 {
          tunnel: [T3 {"Slide Value Low"=0.6, "Slide Value High"=0.7} T3 {"Slide Value Low"=0.65, "Slide Value High"=0.7} T3 {"Slide Value Low"=0.68, "Slide Value High"=0.7}] -> w256
          frame 1, Default {
          }
          frame 2 {
          }
          frame 3 {
          }
        }
        n108 = Bundle By Name(cluster=w257, "Test Info"=w256) -> ()  [unwired: 1 out]
        n109 = call <vilib>:"Add State(s) to Queue__JKI_lib_State_Machine.vi"("State(s) in (\"\")"=w262) -> ("States Out"=w261:string)  [unwired: 14 in]
      }
      frame "LightShow: Set Array Low" {
        # "Your code here.\n(You can make a copy of, or modify, this frame)"
        n110 = local read "Index"() -> (w279:cluster{"Numeric":i32}[][])
        n111 = local read "Array 3"() -> (w288:cluster{"Color Box":u32, "Slide":dbl}[][])
        n112 = Unbundle By Name(w268) -> ("Test Info"=w273:T3)
        n113 = for {
          tunnel: w288 -> [w303] mode=indexing
          tunnel: [w302] -> w272 mode=indexing
          tunnel: [w301] -> w286 mode=indexing
          tunnel: [w300] -> w285 mode=indexing
          tunnel: w279 -> [w299] mode=indexing
          n114 = for {
            tunnel: w303 -> [w306] mode=indexing
            tunnel: [w308] -> w302 mode=indexing
            tunnel: [w308] -> w301 mode=indexing
            tunnel: [w307] -> w300 mode=indexing
            tunnel: w299 -> [w304] mode=indexing
            n115 = Unbundle(w306) -> ("Slide"=w308:dbl)  [unwired: 1 out]
            n116 = Unbundle(w304) -> ("Numeric"=w305:i32)
            n117 = Bundle("Numeric"=w305, "Slide"=w308) -> (w307:cluster{"Numeric":i32, "Slide":dbl})  [unwired: 1 in]
          }
        }
        n118 = Unbundle(w273) -> ("Slide Value Low"=w266:dbl)  [unwired: 1 out]
        n119 = Reshape Array(w285, 36 ("dimension size")) -> (w278:cluster{"Numeric":i32, "Slide":dbl}[])
        n120 = Multiply(x=w266, y=w272) -> (x*y=w271:dbl[][])
        n121 = call "SmartSort.vi"("Array in"=w278) -> ("Array out"=w283:cluster{"Numeric":i32, "Slide":dbl}[])  [unwired: 10 in]
        n122 = call "Voltage to Color.vi"("Array in"=w271) -> ("Array out"=w287:u32[][])  [unwired: 10 in]
        n123 = for {
          N: 32 -> [_]
          tunnel: w283 -> [w292] mode=indexing
          tunnel: [w291] -> w281 mode=indexing
          n124 = Unbundle(w292) -> ("Slide"=w291:dbl)  [unwired: 1 out]
        }
        n125 = local read "physical channels 2"() -> (w275:refnum<k21>)
        n126 = Multiply(x=w266, y=w281) -> (x*y=w280:dbl[])
        n127 = local read "physical channels"() -> (w274:refnum<k21>)
        n128 = Bundle By Name(cluster=w268, "Slide Value"=w266) -> (w267:T4)
        n129 = call "Write to USB Cards.vi"("physical channels"=w275, "physical channels 2"=w274, "Array"=w280, "error in"=w270) -> ("error out"=w276:errorcluster)  [unwired: 5 in]
        n130 = for {
          tunnel: [w293] -> _ mode=indexing
          tunnel: w287 -> [w295] mode=indexing
          tunnel: w286 -> [w294] mode=indexing
          tunnel: [w293] -> w277 mode=indexing
          n131 = for {
            tunnel: [w298] -> w293 mode=indexing
            tunnel: w295 -> [w297] mode=indexing
            tunnel: w294 -> [w296] mode=indexing
            n132 = Bundle(w297, "Slide"=w296) -> (w298:cluster{u32, "Slide":dbl})  [unwired: 1 in]
          }
        }
        n133 = call <vilib>:"Clear Errors.vi"("error in (no error)"=w276) -> ("error out"=w269:errorcluster)  [unwired: 5 in, 1 out]
        n134 = local write "Array 3"(w277) -> ()
        n135 = call <vilib>:"Add State(s) to Queue__JKI_lib_State_Machine.vi"("State(s) in (\"\")"=w290) -> ("States Out"=w289:string)  [unwired: 14 in]
      }
      frame "LightShow: Set Array High" {
        # "Your code here.\n(You can make a copy of, or modify, this frame)"
        n136 = local read "Index"() -> (w322:cluster{"Numeric":i32}[][])
        n137 = local read "Array 3"() -> (w331:cluster{"Color Box":u32, "Slide":dbl}[][])
        n138 = Unbundle By Name(w311) -> ("Test Info"=w316:T3)
        n139 = for {
          tunnel: w331 -> [w346] mode=indexing
          tunnel: [w345] -> w315 mode=indexing
          tunnel: [w344] -> w329 mode=indexing
          tunnel: [w343] -> w328 mode=indexing
          tunnel: w322 -> [w342] mode=indexing
          n140 = for {
            tunnel: w346 -> [w349] mode=indexing
            tunnel: [w351] -> w345 mode=indexing
            tunnel: [w351] -> w344 mode=indexing
            tunnel: [w350] -> w343 mode=indexing
            tunnel: w342 -> [w347] mode=indexing
            n141 = Unbundle(w349) -> ("Slide"=w351:dbl)  [unwired: 1 out]
            n142 = Unbundle(w347) -> ("Numeric"=w348:i32)
            n143 = Bundle("Numeric"=w348, "Slide"=w351) -> (w350:cluster{"Numeric":i32, "Slide":dbl})  [unwired: 1 in]
          }
        }
        n144 = Unbundle(w316) -> ("Slide Value High"=w309:dbl)  [unwired: 1 out]
        n145 = Reshape Array(w328, 36 ("dimension size")) -> (w321:cluster{"Numeric":i32, "Slide":dbl}[])
        n146 = Multiply(x=w309, y=w315) -> (x*y=w314:dbl[][])
        n147 = call "SmartSort.vi"("Array in"=w321) -> ("Array out"=w326:cluster{"Numeric":i32, "Slide":dbl}[])  [unwired: 10 in]
        n148 = call "Voltage to Color.vi"("Array in"=w314) -> ("Array out"=w330:u32[][])  [unwired: 10 in]
        n149 = for {
          N: 32 -> [_]
          tunnel: w326 -> [w335] mode=indexing
          tunnel: [w334] -> w324 mode=indexing
          n150 = Unbundle(w335) -> ("Slide"=w334:dbl)  [unwired: 1 out]
        }
        n151 = local read "physical channels 2"() -> (w318:refnum<k21>)
        n152 = Multiply(x=w309, y=w324) -> (x*y=w323:dbl[])
        n153 = local read "physical channels"() -> (w317:refnum<k21>)
        n154 = Bundle By Name(cluster=w311, "Slide Value"=w309) -> (w310:T4)
        n155 = call "Write to USB Cards.vi"("physical channels"=w318, "physical channels 2"=w317, "Array"=w323, "error in"=w313) -> ("error out"=w319:errorcluster)  [unwired: 5 in]
        n156 = for {
          tunnel: [w336] -> _ mode=indexing
          tunnel: w330 -> [w338] mode=indexing
          tunnel: w329 -> [w337] mode=indexing
          tunnel: [w336] -> w320 mode=indexing
          n157 = for {
            tunnel: [w341] -> w336 mode=indexing
            tunnel: w338 -> [w340] mode=indexing
            tunnel: w337 -> [w339] mode=indexing
            n158 = Bundle(w340, "Slide"=w339) -> (w341:cluster{u32, "Slide":dbl})  [unwired: 1 in]
          }
        }
        n159 = call <vilib>:"Clear Errors.vi"("error in (no error)"=w319) -> ("error out"=w312:errorcluster)  [unwired: 5 in, 1 out]
        n160 = local write "Array 3"(w320) -> ()
        n161 = call <vilib>:"Add State(s) to Queue__JKI_lib_State_Machine.vi"("State(s) in (\"\")"=w333) -> ("States Out"=w332:string)  [unwired: 14 in]
      }
    }
  }
